vi "TempAtTime.vi"(8 "error in (no error)":errorcluster, 10 "theTime":dbl, 11 "thePath":T1) -> (0 "error out":errorcluster, 1 "isValid":bool, 2 "temp":dbl)   [LabVIEW 2012, in "dvotTTPathPoint.lvclass"]
uses:
  dvotTTPathPoint.lvclass
  Controls/TTPath.ctl
panel:
  out "hiPt":i32
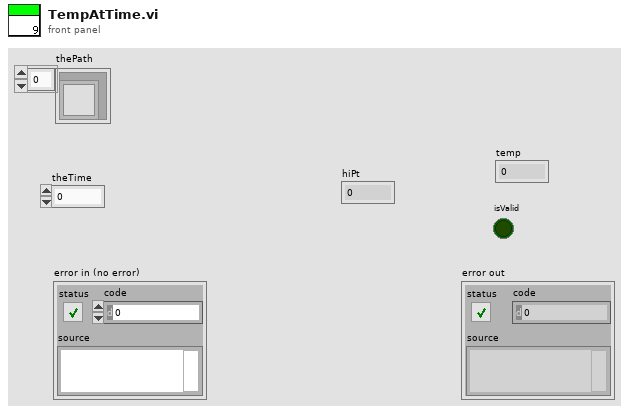
[diagram p1: front panel]
types:
  T1 = typedef "TTPath.ctl" = refnum<class "dvotTTPathPoint.lvclass">[]
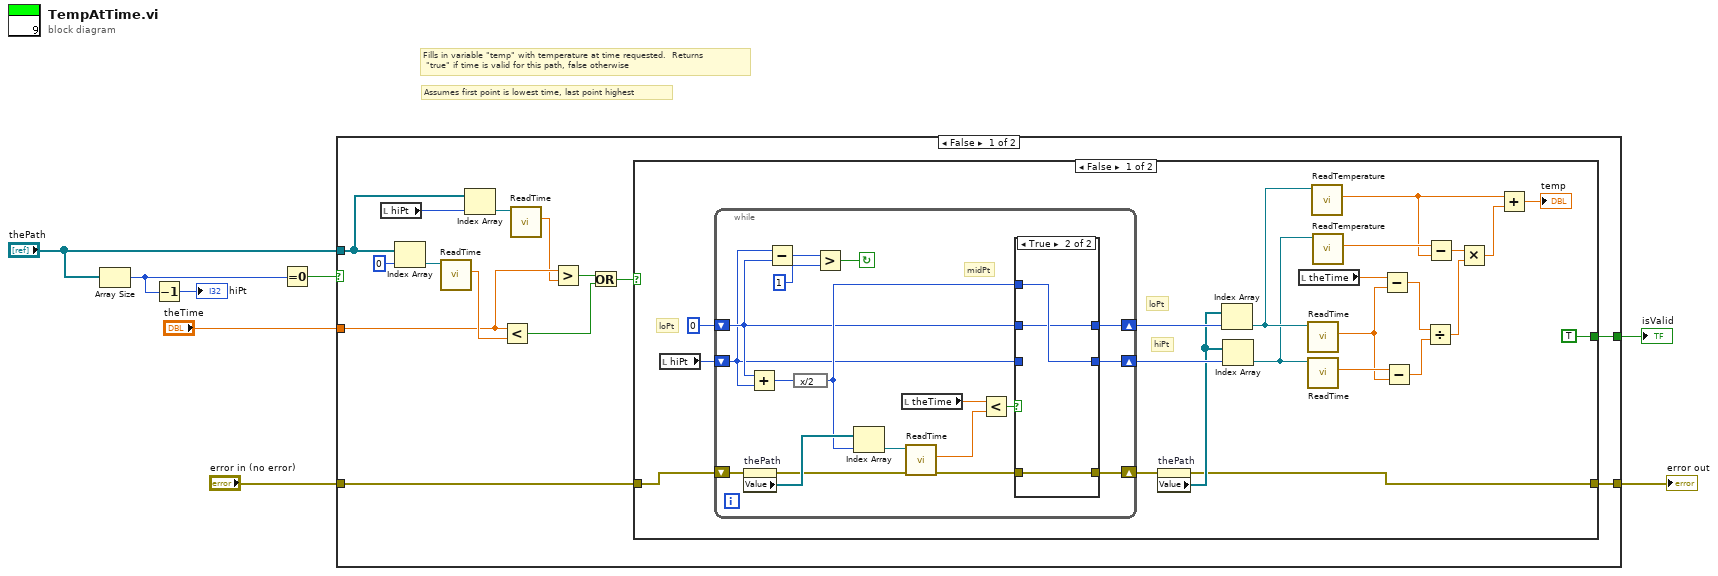
[diagram p0: block diagram]
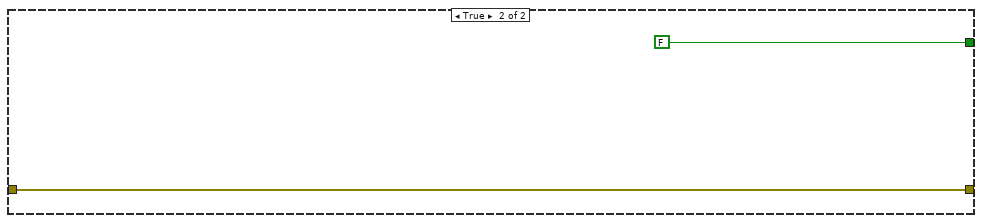
[diagram p3: hidden frame]
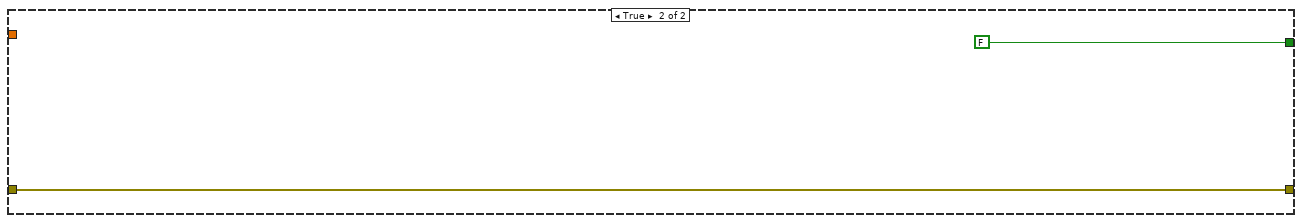
[diagram p4: hidden frame]
diagram:
  # "Assumes first point is lowest time, last point highest"
  # "Fills in variable \"temp\" with temperature at time requested.  Returns\n \"true\" if time is valid for this path, false otherwise"
  n1 = Array Size(array="thePath") -> (size(s)=w2:i32)
  n2 = Decrement(x=w2) -> (x-1=→"hiPt":i32)
  n3 = Equal To 0?(x=w2) -> (x = 0?=w8:bool)
  n4 = case shown="False" w8 {
    tunnel: [w12 FALSE] -> w7
    tunnel: "theTime" -> [w17 _]
    tunnel: "error in (no error)" -> [w10 w71]
    tunnel: "thePath" -> [w19 _]
    tunnel: [w11 w71] -> w3
    frame False {
      n5 = local read "hiPt"() -> (w9:i32)
      n6 = Index Array(array=w19, index=0) -> (element=w22:refnum<class "dvotTTPathPoint.lvclass">)
      n7 = call-dynamic "ReadTime.vi"("dvotTTPathPoint in"=w22) -> ("time"=w18:dbl)  [unwired: 8 in, 2 out]
      n8 = Index Array(array=w19, index=w9) -> (element=w20:refnum<class "dvotTTPathPoint.lvclass">)
      n9 = Less?(x=w17, y=w18) -> (x < y?=w14:bool)
      n10 = call-dynamic "ReadTime.vi"("dvotTTPathPoint in"=w20) -> ("time"=w16:dbl)  [unwired: 8 in, 2 out]
      n11 = Greater?(x=w17, y=w16) -> (0:w15:bool)
      n12 = Or(x=w15, y=w14) -> (x .or. y?=w13:bool)
      n13 = case shown="False" w13 {
        tunnel: [TRUE FALSE] -> w12
        tunnel: [w29 w69] -> w11
        tunnel: w10 -> [w42 w69]
        frame False {
          # "hiPt"
          # "loPt"
          # "loPt"
          n14 = local read "hiPt"() -> (w41:i32)
          n15 = while {
            shift-right: [w49] -> w39
            shift-left: 0 -> [w46]
            shift-right: [w50] -> w38
            shift-left: w41 -> [w45]
            shift-right: [w47] -> w40
            shift-left: w42 -> [w60]
            stop <- w61 continue-if-true
            # "midPt"
            n16 = property on="thePath" class="Arr (strict)"(error in=w60) -> (error out=w55:errorcluster, "Value"=w57:T1)  [unwired: 1 in, 1 out]
            n17 = Add(x=w46, y=w45) -> (x+y=w59:i32)
            n18 = Subtract(x=w45, y=w46) -> (x-y=w52:i32)
            n19 = expression code="x/2"(w59) -> (w51:i32)
            n20 = Greater?(x=w52, y=1) -> (0:w61:bool)
            n21 = Index Array(array=w57, index=w51) -> (element=w56:refnum<class "dvotTTPathPoint.lvclass">)
            n22 = local read "theTime"() -> (w58:dbl)
            n23 = call-dynamic "ReadTime.vi"("error in (no error)"=w55, "dvotTTPathPoint in"=w56) -> ("error out"=w48:errorcluster, "time"=w54:dbl)  [unwired: 7 in, 1 out]
            n24 = Less?(x=w58, y=w54) -> (x < y?=w53:bool)
            n25 = case shown="True" w53 {
              tunnel: w51 -> [w65 w68]
              tunnel: [w63 w68] -> w50
              tunnel: [w65 w66] -> w49
              tunnel: w48 -> [w64 w67]
              tunnel: [w64 w67] -> w47
              tunnel: w46 -> [_ w66]
              tunnel: w45 -> [w63 _]
              frame False {
              }
              frame True {
              }
            }
          }
          n26 = property on="thePath" class="Arr (strict)"(error in=w40) -> (error out=w29:errorcluster, "Value"=w37:T1)  [unwired: 1 in, 1 out]
          n27 = Index Array(array=w37, index=w39) -> (element=w31:refnum<class "dvotTTPathPoint.lvclass">)
          n28 = Index Array(array=w37, index=w38) -> (element=w30:refnum<class "dvotTTPathPoint.lvclass">)
          n29 = local read "theTime"() -> (w36:dbl)
          n30 = call-dynamic "ReadTime.vi"("dvotTTPathPoint in"=w31) -> ("time"=w34:dbl)  [unwired: 8 in, 2 out]
          n31 = call-dynamic "ReadTime.vi"("dvotTTPathPoint in"=w30) -> ("time"=w35:dbl)  [unwired: 8 in, 2 out]
          n32 = call-dynamic "ReadTemperature.vi"("dvotTTPathPoint in"=w31) -> ("temperature"=w27:dbl)  [unwired: 8 in, 2 out]
          n33 = call-dynamic "ReadTemperature.vi"("dvotTTPathPoint in"=w30) -> ("temperature"=w28:dbl)  [unwired: 8 in, 2 out]
          n34 = Subtract(x=w36, y=w34) -> (x-y=w33:dbl)
          n35 = Subtract(x=w35, y=w34) -> (x-y=w32:dbl)
          n36 = Divide(x=w33, y=w32) -> (x/y=w25:dbl)
          n37 = Subtract(x=w28, y=w27) -> (x-y=w26:dbl)
          n38 = Multiply(x=w26, y=w25) -> (x*y=w24:dbl)
          n39 = Add(x=w27, y=w24) -> (x+y=→"temp":dbl)
        }
        frame True {
        }
      }
    }
    frame True {
    }
  }
  "error out" <- w3
  "isValid" <- w7
